vi "lab2_usrp_packet_transceiver.vi"() -> ()   [LabVIEW 2014]
uses:
  <vilib>/addons/Modulation/Analog/support/mod_Set Error Source.vi
  var_stop.vi
  <vilib>/addons/Modulation/Digital/Support/Common/Validators/mod_Generate Filter Coefficients Validate.vi
  <vilib>/addons/Modulation/Digital/General/subVIs/mod_Generate Filter Coefficients.vi
  <vilib>/measure/maspectr.llb/FFT Power Spectrum and PSD for 1 Chan (CDB).vi
  <vilib>/addons/Modulation/Digital/General/MT Apply Matched Filter (Generic).vi
  <vilib>/addons/Modulation/Digital/General/MT Align to Ideal Symbols (Generic).vi
  <instrlib>/niUSRP/niUSRP Fetch Rx Data (CDB Cluster).vi
  <instrlib>/niUSRP/niUSRP Write Tx Data (CDB Cluster).vi
  <vilib>/addons/Modulation/Digital/General/MT Apply Pulse Shaping Filter (Generic).vi
  <vilib>/addons/Modulation/niDMT.lvlib
  <vilib>/measure/NI_MAPro.lvlib
panel:
  out "ser/ber":dbl
  out "received symbols":u32
  out "error symbols":i16
  out "ser":dbl
  out "size2":i32
  out "size1":i32
  out "ber":dbl
  out "received bits":i32
  out "error bits":i16
  out "found?":bool
  out "# elements in queue":i32
  out "Spectrum monitor":cluster{"f0":dbl, "df":dbl, "magnitude":dbl[]}(graph)={"f0"=-0.49993781867926873, "df"=0.00012436264146250465, "magnitude"=[]}
  out "RX Constellation Map":cdb[](graph)
  out "valid?":bool
  in  "Gray code?":bool
  in  "Modulation":enum16{"PSK", "QAM"}(ring)=enum."QAM"
  out "Rx String":string
  in  "String":string
  out "packet len":u32
  in  "Send":bool
  in  "filter length (symbols)":i32=8
  in  "filter parameter":dbl=0.5 format="%.2f"
  in  "pulse shaping filter (none)":T1(ring)=enum."Raised Cosine"
  in  "M-PSK (4)":i32=16 caption="M-ARY"
  in  "samples per symbol (16)":i32=4
  out "packet bits length":i32
  in  "number of samples":i64=40000
  out "RX coerced gain":dbl format="%#_6f"
  out "RX coerced carrier frequency":dbl=915000000.0 format="%#_6p"
  out "RX coerced IQ rate":dbl=4000000.0 format="%#_6p"
  in  "RX active antenna":string="RX2"
  in  "RX gain":dbl format="%#_6f"
  in  "RX device names":refnum<k15>="192.168.10.2"
  out "TX coerced gain":dbl format="%#_6f"
  out "TX coerced carrier frequency":dbl=915000000.0 format="%#_6p"
  out "coerced IQ rate":dbl=4000000.0 format="%#_6p"
  in  "TX device names":refnum<k15>="192.168.10.2"
  in  "TX gain":dbl format="%#_6f"
  in  "carrier frequency":dbl=915000000.0 format="%#_6p"
  in  "IQ rate":dbl=800000.0 format="%#_6p"
  in  "stop":bool
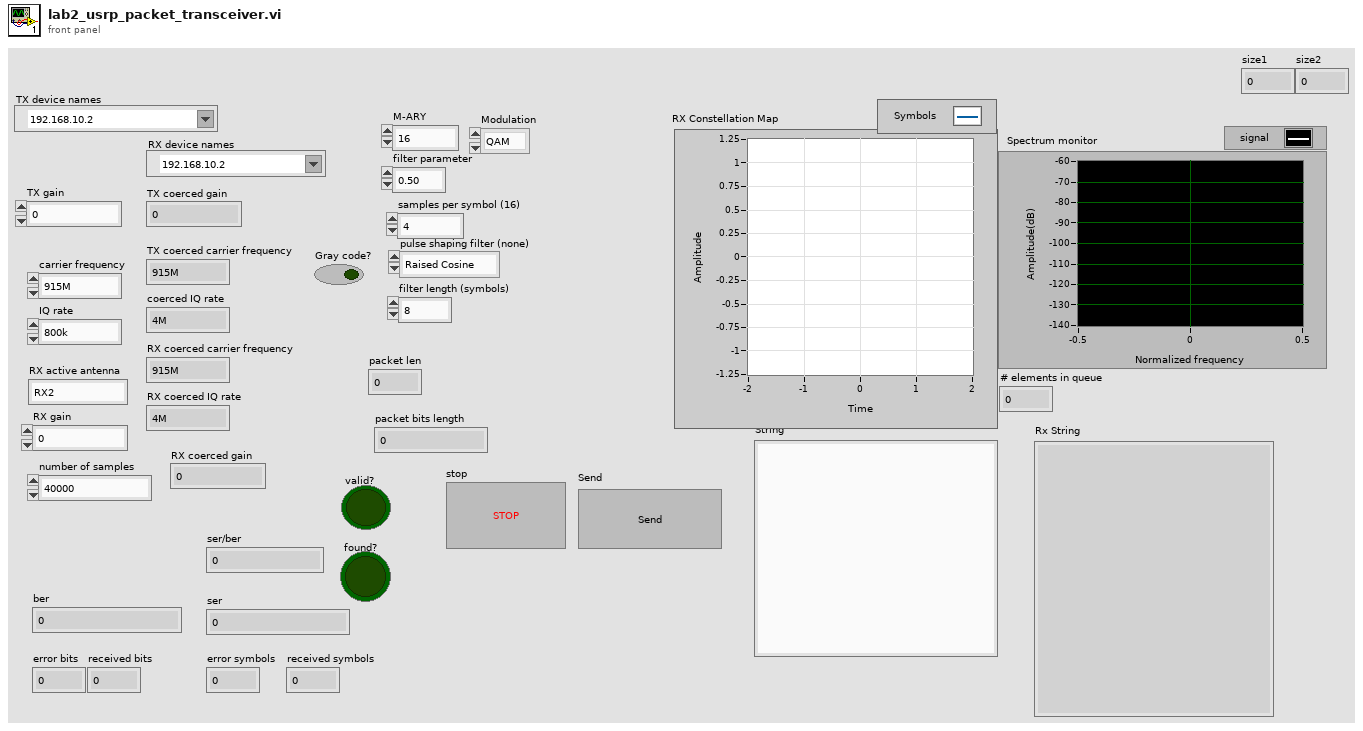
[diagram p1: front panel]
types:
  T1 = enum16{"none", "Raised Cosine", "Root Raised Cos", "Gaussian"}
  T2 = enum16{"FSK", "PSK", "QAM", "MSK", "PAM", "ASK", "CPM"}
  T3 = cluster{"samples per symbol (16)":i32, "symbol map":cdb[], "index map":u32[]}
  T4 = cluster{"samples per symbol (16)":i32, "symbol map":cdb[], i32[]}
  T5 = typedef "niAMT.lvlib/Complex Data Waveform.ctl" = cluster{"t0":dbl, "dt":dbl, "Y":cdb[]}
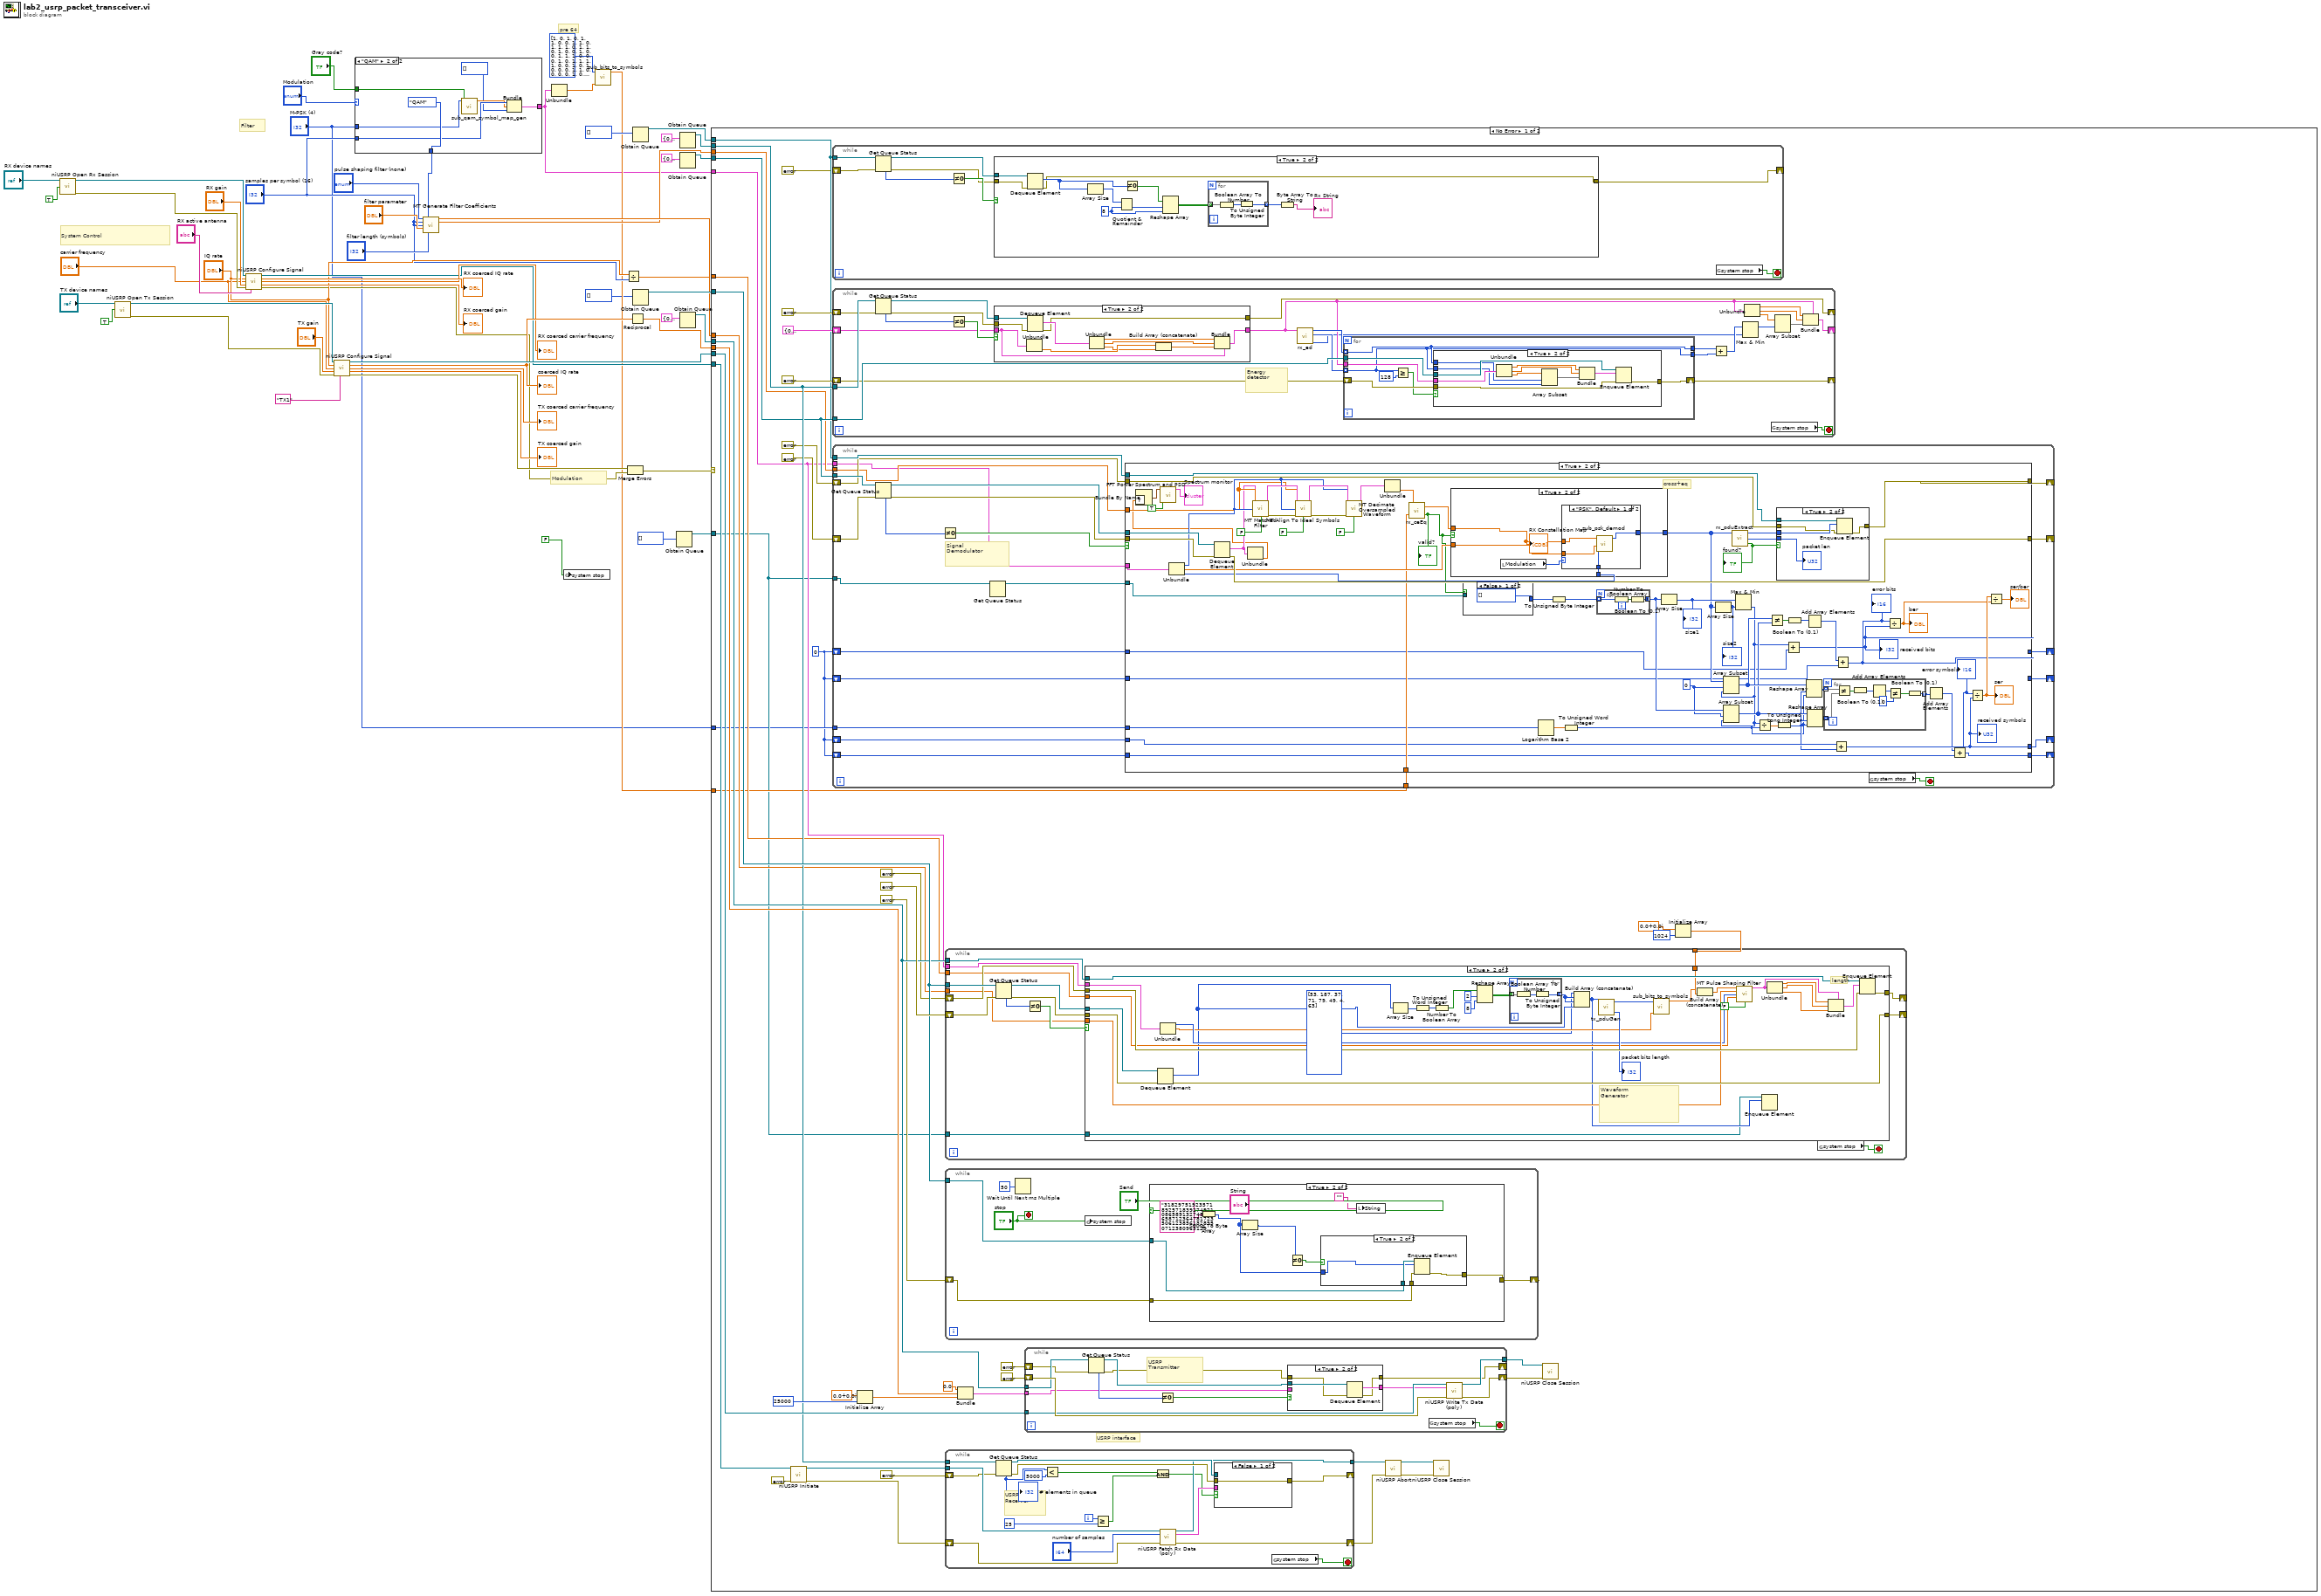
[diagram p0: block diagram]
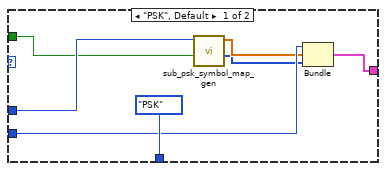
[diagram p2: hidden frame]
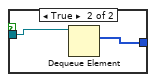
[diagram p5: hidden frame]
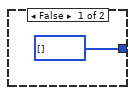
[diagram p6: hidden frame]
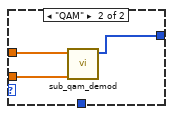
[diagram p7: hidden frame]
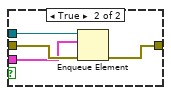
[diagram p11: hidden frame]
diagram:
  # "pre 64"
  # "Modulation"
  # "Filter"
  # "System Control"
  n1 = call <instrlib>:"niUSRP Open Rx Session.vi"("device names"="RX device names", "reset"=TRUE) -> ("session handle out"=w40:refnum<k15>, "error out"=w39:errorcluster)  [unwired: 12 in]
  n2 = call <instrlib>:"niUSRP Open Tx Session.vi"("device names"="TX device names", "reset"=TRUE) -> ("session handle out"=w53:refnum<k15>, "error out"=w52:errorcluster)  [unwired: 12 in]
  n3 = call <instrlib>:"niUSRP Configure Signal.vi"("session handle"=w40, "IQ rate"="IQ rate", "carrier frequency"="carrier frequency", "gain"="RX gain", "error in (no error)"=w39, "active antenna"="RX active antenna") -> ("session handle out"=w31:refnum<k15>, "coerced IQ rate"=→"RX coerced IQ rate":dbl, "coerced carrier frequency"=→"RX coerced carrier frequency":dbl, "coerced gain"=→"RX coerced gain":dbl, "error out"=w15:errorcluster)  [unwired: 5 in]
  n4 = call <instrlib>:"niUSRP Configure Signal.vi"("session handle"=w53, "IQ rate"="IQ rate", "carrier frequency"="carrier frequency", "gain"="TX gain", "error in (no error)"=w52, "active antenna"="TX1") -> ("session handle out"=w44:refnum<k15>, "coerced IQ rate"=w42:dbl, "coerced carrier frequency"=→"TX coerced carrier frequency":dbl, "coerced gain"=→"TX coerced gain":dbl, "error out"=w16:errorcluster)  [unwired: 5 in]
  "coerced IQ rate" <- w42
  n5 = case shown="\"QAM\"" "Modulation" {
    tunnel: [T2."PSK" ("modulation type") T2."QAM" ("modulation type")] -> w11
    tunnel: "M-PSK (4)" -> [w60 w66]
    tunnel: "Gray code?" -> [w59 w67]
    tunnel: "samples per symbol (16)" -> [w58 w65]
    tunnel: [w55 w62] -> w5
    frame "PSK", Default {
      n6 = call "sub_psk_symbol_map_gen.vi"("Gray code?"=w59, "M-PSK"=w60) -> ("index map"=w56:u32[], "symbol map"=w57:cdb[])  [unwired: 8 in]
      n7 = Bundle("samples per symbol (16)"=w58, "symbol map"=w57, "index map"=w56) -> (w55:T3)  [unwired: 1 in]
    }
    frame "QAM" {
      n8 = call "sub_qam_symbol_map_gen.vi"("Gray code?"=w67, "M-QAM"=w66) -> ("symbol map"=w64:cdb[])  [unwired: 9 in]
      n9 = Bundle("samples per symbol (16)"=w65, "symbol map"=w64, i32[] []) -> (w62:T4)  [unwired: 1 in]
    }
  }
  n10 = call <vilib>:"MT Generate Filter Coefficients.vi"("pulse shaping filter (none)"="pulse shaping filter (none)", "modulation type"=w11, "pulse shaping samples per symbol (16)"="samples per symbol (16)", "matched samples per symbol (16)"="samples per symbol (16)", "filter parameter"="filter parameter", "filter length (symbols)"="filter length (symbols)") -> ("pulse shaping filter coefficients"=w21:dbl[], "matched filter coefficients"=w19:dbl[])  [unwired: 7 in, 1 out]
  n11 = Unbundle(w5) -> ("symbol map"=w7:cdb[])  [unwired: 2 out]
  n12 = global write "var_stop.vi" "system stop"(FALSE) -> ()
  n13 = call "sub_bits_to_symbols.vi"("symbol map"=w7, "bits"=i16[] [1, 0, 1, 0, 1, 1, 0, 0, 1, 1, 0, 1, 1, 1, 0, 1, 1, 0, 1, 0, 0, 1, 0, 0, 1, 1, 1, 0, 0, 0, 1, 0, 1, 1, 1, 1, 0, 0, 1, 0, 1, 0, 0, 0, 1, 1, 0, 0, 0, 0, 1, 0, 0, 0, 0, 0, 1, 1, 1, 1, 1, 1, 0, 0] ("preamble(64) 2")) -> ("symbols"=w6:cdb[])  [unwired: 9 in]
  n14 = Divide(x="IQ rate", y="samples per symbol (16)") -> (x/y=w20:dbl)
  n15 = Merge Errors(w16, w15) -> (w14:errorcluster)
  n16 = Reciprocal(x=w42) -> (1/x=w41:dbl)
  n17 = Obtain Queue(element data type=i8[] [] ("output bit stream")) -> (queue out=w26:refnum<queue>)  [unwired: 4 in, 2 out]
  n18 = Obtain Queue(element data type=i16[] []) -> (queue out=w54:refnum<queue>)  [unwired: 4 in, 2 out]
  n19 = Obtain Queue(element data type=i16[] []) -> (queue out=w2:refnum<queue>)  [unwired: 4 in, 2 out]
  n20 = Obtain Queue(element data type=cluster{"t0":dbl, "dt":dbl, "Y":cdb[]} {"t0"=0.0, "dt"=0.0, "Y"=[]} ("data")) -> (queue out=w30:refnum<queue>)  [unwired: 4 in, 2 out]
  n21 = Obtain Queue(element data type=cluster{"t0":dbl, "dt":dbl, "Y":cdb[]} {"t0"=0.0, "dt"=0.0, "Y"=[]} ("data")) -> (queue out=w27:refnum<queue>)  [unwired: 4 in, 2 out]
  n22 = Obtain Queue(element data type=cluster{"t0":dbl, "dt":dbl, "Y":cdb[]} {"t0"=0.0, "dt"=1.0, "Y"=[]} ("data")) -> (queue out=w45:refnum<queue>)  [unwired: 4 in, 2 out]
  n23 = case shown="No Error" w14 {
    tunnel: w54 -> [w112 _]
    tunnel: w45 -> [w107 _]
    tunnel: w44 -> [w108 _]
    tunnel: w41 -> [w101 _]
    tunnel: w31 -> [w96 _]
    tunnel: w30 -> [w90 _]
    tunnel: w27 -> [w86 _]
    tunnel: w26 -> [w84 _]
    tunnel: w5 -> [w78 _]
    tunnel: w21 -> [w81 _]
    tunnel: w20 -> [w80 _]
    tunnel: w19 -> [w79 _]
    tunnel: w6 -> [w72 _]
    tunnel: w2 -> [w71 _]
    tunnel: "M-PSK (4)" -> [w70 _]
    frame No Error {
      w69 = 0
      # "USRP interface"
      n24 = call <instrlib>:"niUSRP Initiate.vi"("session handle"=w96, "error in (no error)"=errorcluster {"status"=FALSE, "code"=0, "source"=""}) -> ("session handle out"=w95:refnum<k15>, "error out"=w94:errorcluster)  [unwired: 12 in]
      n25 = while {
        tunnel: w84 -> [w121]
        shift-right: [w114] -> _
        shift-left: errorcluster {"status"=FALSE, "code"=0, "source"=""} ("error out") -> [w120]
        stop <- w119 stop-if-true
        n26 = Get Queue Status(queue=w121, error in (no error)=w120) -> (queue out=w116:refnum<queue>, error out=w115:errorcluster, # elements in queue=w118:i32)  [unwired: 1 in, 5 out]
        n27 = Not Equal To 0?(x=w118) -> (x != 0?=w117:bool)
        n28 = case shown="True" w117 {
          tunnel: w116 -> [_ w133]
          tunnel: w115 -> [w122 w132]
          tunnel: [w122 w125] -> w114
          frame False {
          }
          frame True {
            w128 = 8 ("y")
            n29 = Dequeue Element(queue=w133, error in (no error)=w132) -> (element=w131:i8[], error out=w125:errorcluster)  [unwired: 1 in, 2 out]
            n30 = Array Size(array=w131) -> (size(s)=w130:i32)
            n31 = Quotient & Remainder(x=w130, y=w128) -> (floor(x/y)=w127:i32)  [unwired: 1 out]
            n32 = Not Equal To 0?(x=w131) -> (x != 0?=w129:bool[])
            n33 = Reshape Array(w129, w127, w128) -> (w126:bool[][])
            n34 = for {
              tunnel: w126 -> [w136] mode=indexing
              tunnel: [w135] -> w124 mode=indexing
              n35 = Boolean Array To Number(Boolean array=w136) -> (number=w134:u32)
              n36 = To Unsigned Byte Integer(number=w134) -> (unsigned 8bit integer=w135:u8)
            }
            n37 = Byte Array To String(unsigned byte array=w124) -> (string=→"Rx String":string)
          }
        }
        n38 = global read "var_stop.vi" "system stop"() -> (w119:bool)
      }
      n39 = while {
        tunnel: w90 -> [w290]
        shift-right: [w283] -> _
        shift-left: errorcluster {"status"=FALSE, "code"=0, "source"=""} ("error out") -> [w289]
        shift-right: [w269] -> _
        shift-left: cluster{"t0":dbl, "dt":dbl, "Y":cdb[]} {"t0"=0.0, "dt"=0.0, "Y"=[]} ("data") -> [w284]
        tunnel: w86 -> [w282]
        shift-right: [w281] -> _
        shift-left: errorcluster {"status"=FALSE, "code"=0, "source"=""} ("error out") -> [w280]
        stop <- w279 stop-if-true
        # "Energy\ndetector"
        n40 = Get Queue Status(queue=w290, error in (no error)=w289) -> (queue out=w285:refnum<queue>, error out=w286:errorcluster, # elements in queue=w288:i32)  [unwired: 1 in, 5 out]
        n41 = Not Equal To 0?(x=w288) -> (x != 0?=w287:bool)
        n42 = case shown="True" w287 {
          tunnel: w286 -> [w312 w323]
          tunnel: w285 -> [_ w322]
          tunnel: w284 -> [w311 w317]
          tunnel: [w312 w314] -> w283
          tunnel: [w311 w313] -> w276
          frame False {
          }
          frame True {
            n43 = Unbundle(w317) -> ("Y"=w320:cdb[])  [unwired: 2 out]
            n44 = Dequeue Element(queue=w322, error in (no error)=w323) -> (element=w321:cluster{"t0":dbl, "dt":dbl, "Y":cdb[]}, error out=w314:errorcluster)  [unwired: 1 in, 2 out]
            n45 = Unbundle(w321) -> ("t0"=w316:dbl, "dt"=w315:dbl, "Y"=w319:cdb[])
            n46 = Build Array (concatenate)(w320, w319) -> (w318:cdb[])
            n47 = Bundle(cluster=w317, "t0"=w316, "dt"=w315, "Y"=w318) -> (w313:cluster{"t0":dbl, "dt":dbl, "Y":cdb[]})
          }
        }
        n48 = call "rx_ed.vi"("Wavefrom"=w276) -> ("first pulse"=w266:i32, "length"=w277:i32[], "start index"=w278:i32[])  [unwired: 8 in]
        n49 = for {
          tunnel: w282 -> [w298]
          tunnel: w276 -> [w295]
          shift-right: [w297] -> w281
          shift-left: w280 -> [w296]
          tunnel: w278 -> [w294] mode=indexing
          tunnel: w277 -> [w293] mode=indexing
          tunnel: [w294] -> w272
          tunnel: [w293] -> w271
          n50 = Greater Or Equal?(x=w293, y=128) -> (x >= y?=w291:bool)
          n51 = case shown="True" w291 {
            tunnel: w298 -> [_ w310]
            tunnel: [w299 w309] -> w297
            tunnel: w296 -> [w299 w308]
            tunnel: w295 -> [_ w307]
            tunnel: w294 -> [_ w301]
            tunnel: w293 -> [_ w300]
            frame False {
            }
            frame True {
              n52 = Unbundle(w307) -> ("t0"=w305:dbl, "dt"=w306:dbl, "Y"=w303:cdb[])
              n53 = Array Subset(array=w303, index=w301, length=w300) -> (w302:cdb[])
              n54 = Bundle("t0"=w305, "dt"=w306, w302) -> (w304:cluster{"t0":dbl, "dt":dbl, cdb[]})  [unwired: 1 in]
              n55 = Enqueue Element(queue=w310, element=w304, error in (no error)=w308) -> (error out=w309:errorcluster)  [unwired: 1 in, 2 out]
            }
          }
        }
        n56 = Add(x=w272, y=w271) -> (x+y=w268:i32)
        n57 = Max & Min(x=w268, y=w266) -> (max(x,y)=w267:i32)  [unwired: 1 out]
        n58 = Unbundle(w276) -> ("t0"=w275:dbl, "dt"=w274:dbl, "Y"=w273:cdb[])
        n59 = global read "var_stop.vi" "system stop"() -> (w279:bool)
        n60 = Array Subset(array=w273, index=w267) -> (w270:cdb[])  [unwired: 1 in]
        n61 = Bundle(cluster=w276, "t0"=w275, "dt"=w274, "Y"=w270) -> (w269:cluster{"t0":dbl, "dt":dbl, "Y":cdb[]})
      }
      n62 = while {
        tunnel: w86 -> [w161]
        shift-right: [w155] -> _
        shift-left: errorcluster {"status"=FALSE, "code"=0, "source"=""} ("error out") -> [w160]
        tunnel: w84 -> [w154]
        shift-right: [w153] -> _
        shift-left: errorcluster {"status"=FALSE, "code"=0, "source"=""} ("error out") -> [w152]
        tunnel: w79 -> [w150]
        tunnel: w78 -> [w149]
        tunnel: w72 -> [w148]
        tunnel: w71 -> [w147]
        tunnel: w70 -> [w145]
        shift-right: [w142] -> _
        shift-left: w69 -> [w144]
        shift-right: [w141] -> _
        shift-left: w69 -> [w143]
        shift-right: [w139] -> _
        shift-left: w69 -> [w140]
        shift-right: [w137] -> _
        shift-left: w69 -> [w138]
        stop <- w151 stop-if-true
        # "Signal \nDemodulator"
        n63 = Get Queue Status(queue=w161, error in (no error)=w160) -> (queue out=w157:refnum<queue>, error out=w156:errorcluster, # elements in queue=w159:i32)  [unwired: 1 in, 5 out]
        n64 = Not Equal To 0?(x=w159) -> (x != 0?=w158:bool)
        n65 = Get Queue Status(queue=w147) -> (queue out=w146:refnum<queue>)  [unwired: 2 in, 7 out]
        n66 = case shown="True" w158 {
          tunnel: w157 -> [_ w231]
          tunnel: w156 -> [w167 w232]
          tunnel: [w167 w230] -> w155
          tunnel: w154 -> [_ w221]
          tunnel: [w166 w220] -> w153
          tunnel: w152 -> [w166 w219]
          tunnel: w150 -> [_ w209]
          tunnel: w149 -> [_ w213]
          tunnel: w148 -> [_ w205]
          tunnel: w146 -> [_ w173]
          tunnel: w145 -> [_ w170]
          tunnel: w144 -> [w165 w184]
          tunnel: w143 -> [w164 w183]
          tunnel: [w165 w174] -> w142
          tunnel: [w164 w181] -> w141
          tunnel: w140 -> [w163 w180]
          tunnel: [w163 w178] -> w139
          tunnel: w138 -> [w162 w177]
          tunnel: [w162 w175] -> w137
          frame False {
          }
          frame True {
            w197 = 0
            # "cross+eq"
            n67 = Unbundle(w213) -> ("samples per symbol (16)"=w212:i32, "symbol map"=w211:cdb[], "index map"=w210:u32[])
            n68 = Dequeue Element(queue=w231, error in (no error)=w232) -> (element=w204:cluster{"t0":dbl, "dt":dbl, "Y":cdb[]}, error out=w230:errorcluster)  [unwired: 1 in, 2 out]
            n69 = Unbundle(w204) -> ("Y"=w203:cdb[])  [unwired: 2 out]
            n70 = Bundle By Name("Y"=w203) -> (w208:waveform(cdb))  [unwired: 1 in]
            n71 = call-poly <vilib>:"FFT Power Spectrum and PSD.vi"("dB On (F)"=TRUE, "time signal"=w208) -> ("Power Spectrum / PSD"=→"Spectrum monitor":cluster{"f0":dbl, "df":dbl, "magnitude":dbl[]})  [unwired: 6 in, 3 out]
            n72 = call-poly <vilib>:"MT Matched Filter.vi"("input complex waveform"=w204, "matched filter coefficients"=w209, "samples per symbol (16)"=w212, "reset? (T)"=FALSE) -> ("output complex waveform"=w229:T5, "error out"=w228:errorcluster)  [unwired: 10 in]
            n73 = call-poly <vilib>:"MT Align To Ideal Symbols.vi"("input complex waveform"=w229, "matched filter coefficients"=w209, "samples per symbol (16)"=w212, "error in (no error)"=w228, "reset? (T)"=FALSE) -> ("output complex waveform"=w226:T5, "error out"=w227:errorcluster)  [unwired: 8 in, 1 out]
            n74 = call <vilib>:"MT Decimate Oversampled Waveform.vi"("input complex waveform"=w226, "decimation factor"=w212, "error in (no error)"=w227, "reset? (T)"=FALSE) -> ("output complex waveform"=w225:T5)  [unwired: 10 in, 1 out]
            n75 = Unbundle(w225) -> ("Y"=w222:cdb[])  [unwired: 2 out]
            n76 = call "rx_ceEq.vi"("preamble"=w205, "symbols"=w222) -> ("valid?"=w171:bool, "eq symbols"=w218:cdb[])
            "valid?" <- w171
            n77 = case shown="True" w171 {
              tunnel: [i8[] [] ("output bit stream") w250] -> w199
              tunnel: w211 -> [_ w251]
              tunnel: w218 -> [_ w248]
              tunnel: w210 -> [_ w249]
              frame False {
              }
              frame True {
                n78 = local read "Modulation"() -> (w252:enum16{"PSK", "QAM"})
                n79 = case shown="\"PSK\", Default" w252 {
                  tunnel: w248 -> [w256 w259]
                  tunnel: w251 -> [w255 w258]
                  tunnel: [w253 w257] -> w250
                  tunnel: w249 -> [w254 _]
                  frame "PSK", Default {
                    n80 = call "sub_psk_demod.vi"("index map"=w254, "symbol map"=w255, "symbol"=w256) -> ("bitstream"=w253:i16[])  [unwired: 8 in]
                  }
                  frame "QAM" {
                    n81 = call "sub_qam_demod.vi"("symbol map"=w258, "symbol"=w259) -> ("bitstream"=w257:i16[])  [unwired: 9 in]
                  }
                }
                "RX Constellation Map" <- w248
              }
            }
            n82 = case shown="False" w171 {
              tunnel: w173 -> [_ w235]
              tunnel: [u16[] [] w234] -> w172
              frame False {
              }
              frame True {
                n83 = Dequeue Element(queue=w235) -> (element=w234:i16[])  [unwired: 2 in, 3 out]
              }
            }
            n84 = Logarithm Base 2(1:w170) -> (0:w169:dbl)
            n85 = To Unsigned Byte Integer(number=w172) -> (unsigned 8bit integer=w200:u8[])
            n86 = To Unsigned Word Integer(number=w169) -> (unsigned 16bit integer=w168:u16)
            n87 = for {
              tunnel: w200 -> [w246] mode=indexing
              tunnel: [w244] -> w198 mode=concatenating
              n88 = Number To Boolean Array(number=w246) -> (Boolean array=w245:bool[])
              n89 = Boolean To (0,1)(Boolean=w245) -> (0, 1=w244:i16[])
            }
            n90 = Array Size(array=w198) -> (size(s)=w201:i32)
            "size1" <- w201
            n91 = Array Size(array=w199) -> (size(s)=w202:i32)
            "size2" <- w202
            n92 = call "rx_pduExtract.vi"("output bit stream"=w199) -> ("found?"=w224:bool, "packet len"=w217:u32, "ppdu"=w223:i8[])  [unwired: 2 in]
            "found?" <- w224
            n93 = Max & Min(x=w201, y=w202) -> (min(x,y)=w185:i32)  [unwired: 1 out]
            n94 = Array Subset(array=w199, index=w197, length=w185) -> (w194:i16[])
            n95 = Array Subset(array=w198, index=w197, length=w185) -> (w193:i16[])
            n96 = Divide(x=w185, y=w168) -> (x/y=w189:dbl)
            n97 = Not Equal?(x=w194, y=w193) -> (x != y?=w196:bool[])
            n98 = case shown="True" w224 {
              tunnel: w223 -> [_ w263]
              tunnel: w221 -> [_ w265]
              tunnel: [w260 w264] -> w220
              tunnel: w219 -> [w260 w261]
              tunnel: w217 -> [_ w262]
              frame False {
              }
              frame True {
                n99 = Enqueue Element(queue=w265, element=w263, error in (no error)=w261) -> (error out=w264:errorcluster)  [unwired: 1 in, 2 out]
                "packet len" <- w262
              }
            }
            n100 = To Unsigned Long Integer(number=w189) -> (unsigned 32bit integer=w179:u32)
            n101 = Add(x=w185, y=w184) -> (x+y=w174:i32)
            "received bits" <- w174
            n102 = Boolean To (0,1)(Boolean=w196) -> (0, 1=w195:i16[])
            n103 = Reshape Array(w194, w179, w168) -> (w192:i16[][])
            n104 = Add Array Elements(numeric array=w195) -> (sum=w182:i16)
            n105 = Reshape Array(w193, w179, w168) -> (w191:i16[][])
            n106 = for {
              tunnel: w192 -> [w238] mode=indexing
              tunnel: w191 -> [w237] mode=indexing
              tunnel: [w236] -> w190 mode=indexing
              n107 = Not Equal?(x=w238, y=w237) -> (x != y?=w243:bool[])
              n108 = Boolean To (0,1)(Boolean=w243) -> (0, 1=w242:i16[])
              n109 = Add Array Elements(numeric array=w242) -> (sum=w241:i16)
              n110 = Not Equal?(x=w241, y=0) -> (x != y?=w239:bool)
              n111 = Boolean To (0,1)(Boolean=w239) -> (0, 1=w236:i16)
            }
            n112 = Add(x=w180, y=w179) -> (x+y=w178:u32)
            "received symbols" <- w178
            n113 = Add(x=w182, y=w183) -> (x+y=w181:i32)
            "error bits" <- w181
            n114 = Divide(x=w181, y=w174) -> (x/y=w187:dbl)
            "ber" <- w187
            n115 = Add Array Elements(numeric array=w190) -> (sum=w176:i16)
            n116 = Add(x=w176, y=w177) -> (x+y=w175:i32)
            "error symbols" <- w175
            n117 = Divide(x=w175, y=w178) -> (x/y=w188:dbl)
            "ser" <- w188
            n118 = Divide(x=w188, y=w187) -> (x/y=→"ser/ber":dbl)
          }
        }
        n119 = global read "var_stop.vi" "system stop"() -> (w151:bool)
      }
      n120 = Initialize Array(cdb 0.0+0.0i, 25000 ("dimension size")) -> (w102:cdb[])
      n121 = while {
        tunnel: w112 -> [w425]
        shift-right: [w423] -> _
        shift-left: errorcluster {"status"=FALSE, "code"=0, "source"=""} ("error out") -> [w424]
        stop <- "stop" stop-if-true
        n122 = Wait Until Next ms Multiple(millisecond multiple=u32 50) -> ()  [unwired: 1 out]
        n123 = global write "var_stop.vi" "system stop"("stop") -> ()
        n124 = case shown="True" "Send" {
          tunnel: w425 -> [_ w433]
          tunnel: w424 -> [w428 w432]
          tunnel: [w428 w431] -> w423
          frame False {
          }
          frame True {
            n125 = String To Byte Array(string="318297519235718925718392749210865891327481326587123647817235061238561328950712380965129083740123658129379123658291374931829751923571892571839274921086589132748132658712364781723506123856132895071238096512908374012365812937912365829137493182975192357189257183927492108658913274813265871236478172350612385613289507123809651290837401236581293791236582913749") -> (unsigned byte array=w434:u8[])
            n126 = Array Size(array=w434) -> (size(s)=w430:i32)
            n127 = Not Equal To 0?(x=w430) -> (x != 0?=w435:bool)
            n128 = case shown="True" w435 {
              tunnel: w434 -> [_ w438]
              tunnel: w433 -> [_ w441]
              tunnel: w432 -> [w437 w440]
              tunnel: [w437 w439] -> w431
              frame False {
              }
              frame True {
                n129 = Enqueue Element(queue=w441, element=w438, error in (no error)=w440) -> (error out=w439:errorcluster)  [unwired: 1 in, 2 out]
              }
            }
            n130 = local write "String"("") -> ()
          }
        }
      }
      n131 = while {
        tunnel: w95 -> [w342]
        shift-right: [w330] -> w91
        shift-left: w94 -> [w341]
        tunnel: w90 -> [w339]
        shift-right: [w333] -> _
        shift-left: errorcluster {"status"=FALSE, "code"=0, "source"=""} ("error out") -> [w338]
        tunnel: [w331] -> w92
        i -> [w328]
        stop <- w329 stop-if-true
        # "USRP\nReceiver"
        n132 = Get Queue Status(queue=w339, error in (no error)=w338) -> (queue out=w335:refnum<queue>, error out=w334:errorcluster, # elements in queue=w337:i32)  [unwired: 1 in, 5 out]
        "# elements in queue" <- w337
        n133 = Less?(x=w337, y=5000) -> (x < y?=w326:bool)
        n134 = Greater Or Equal?(x=w328, y=25) -> (x >= y?=w325:bool)
        n135 = And(x=w326, y=w325) -> (x .and. y?=w324:bool)
        n136 = call-poly <instrlib>:"niUSRP Fetch Rx Data (poly).vi"("session handle"=w342, "number of samples"="number of samples", "error in (no error)"=w341) -> ("session handle out"=w331:refnum<k15>, "data"=w332:cluster{"t0":dbl, "dt":dbl, "Y":cdb[]}, "error out"=w330:errorcluster)  [unwired: 9 in, 1 out]
        n137 = case shown="False" w324 {
          tunnel: w335 -> [_ w347]
          tunnel: w334 -> [w343 w346]
          tunnel: [w343 w345] -> w333
          tunnel: w332 -> [_ w344]
          frame False {
          }
          frame True {
            n138 = Enqueue Element(queue=w347, element=w344, error in (no error)=w346) -> (error out=w345:errorcluster)  [unwired: 1 in, 2 out]
          }
        }
        n139 = global read "var_stop.vi" "system stop"() -> (w329:bool)
      }
      n140 = Bundle(0.0, w101, w102) -> (w99:cluster{dbl, dbl, cdb[]})  [unwired: 1 in]
      n141 = while {
        shift-right: [w357] -> w111
        shift-left: errorcluster {"status"=FALSE, "code"=0, "source"=""} ("error out") -> [w355]
        tunnel: [w356] -> w110
        tunnel: w108 -> [w354]
        tunnel: w107 -> [w352]
        shift-right: [w350] -> _
        shift-left: errorcluster {"status"=FALSE, "code"=0, "source"=""} ("error out") -> [w351]
        tunnel: w99 -> [w349]
        stop <- w348 stop-if-true
        # "USRP\nTransmitter"
        n142 = Get Queue Status(queue=w352, error in (no error)=w351) -> (queue out=w359:refnum<queue>, error out=w358:errorcluster, # elements in queue=w361:i32)  [unwired: 1 in, 5 out]
        n143 = Not Equal To 0?(x=w361) -> (x != 0?=w360:bool)
        n144 = case shown="True" w360 {
          tunnel: w359 -> [_ w367]
          tunnel: w358 -> [w362 w366]
          tunnel: [w363 w365] -> w353
          tunnel: [w362 w364] -> w350
          tunnel: w349 -> [w363 _]
          frame False {
          }
          frame True {
            n145 = Dequeue Element(queue=w367, error in (no error)=w366) -> (element=w365:cluster{"t0":dbl, "dt":dbl, "Y":cdb[]}, error out=w364:errorcluster)  [unwired: 1 in, 2 out]
          }
        }
        n146 = global read "var_stop.vi" "system stop"() -> (w348:bool)
        n147 = call-poly <instrlib>:"niUSRP Write Tx Data (poly).vi"("session handle"=w354, "data"=w353, "error in (no error)"=w355) -> ("session handle out"=w356:refnum<k15>, "error out"=w357:errorcluster)  [unwired: 11 in]
      }
      n148 = call <instrlib>:"niUSRP Abort.vi"("session handle"=w92, "error in (no error)"=w91) -> ("session handle out"=w98:refnum<k15>, "error out"=w97:errorcluster)  [unwired: 12 in]
      n149 = call <instrlib>:"niUSRP Close Session.vi"("session handle"=w98, "error in (no error)"=w97) -> ()  [unwired: 13 in, 1 out]
      n150 = call <instrlib>:"niUSRP Close Session.vi"("session handle"=w110, "error in (no error)"=w111) -> ()  [unwired: 13 in, 1 out]
      n151 = Initialize Array(cdb 0.0+0.0i, 1024 ("dimension size")) -> (w73:cdb[])
      n152 = while {
        tunnel: w112 -> [w380]
        shift-right: [w377] -> _
        shift-left: errorcluster {"status"=FALSE, "code"=0, "source"=""} ("error out") -> [w383]
        tunnel: w107 -> [w376]
        shift-right: [w375] -> _
        shift-left: errorcluster {"status"=FALSE, "code"=0, "source"=""} ("error out") -> [w374]
        tunnel: w78 -> [w372]
        tunnel: w81 -> [w371]
        tunnel: w80 -> [w370]
        tunnel: w73 -> [w369]
        tunnel: w71 -> [w368]
        stop <- w373 stop-if-true
        n153 = Get Queue Status(queue=w380, error in (no error)=w383) -> (queue out=w378:refnum<queue>, error out=w379:errorcluster, # elements in queue=w382:i32)  [unwired: 1 in, 5 out]
        n154 = Not Equal To 0?(x=w382) -> (x != 0?=w381:bool)
        n155 = case shown="True" w381 {
          tunnel: w379 -> [w385 w418]
          tunnel: w378 -> [_ w417]
          tunnel: [w385 w416] -> w377
          tunnel: w376 -> [_ w411]
          tunnel: [w384 w410] -> w375
          tunnel: w374 -> [w384 w409]
          tunnel: w372 -> [_ w407]
          tunnel: w371 -> [_ w406]
          tunnel: w370 -> [_ w405]
          tunnel: w369 -> [_ w395]
          tunnel: w368 -> [_ w386]
          frame False {
          }
          frame True {
            # "length"
            # "Waveform \nGenerator"
            n156 = Dequeue Element(queue=w417, error in (no error)=w418) -> (element=w391:i16[], error out=w416:errorcluster)  [unwired: 1 in, 2 out]
            n157 = Unbundle(w407) -> ("samples per symbol (16)"=w401:i32, "symbol map"=w393:cdb[])  [unwired: 1 out]
            n158 = Array Size(array=w391) -> (size(s)=w403:i32)
            n159 = To Unsigned Word Integer(number=w403) -> (unsigned 16bit integer=w402:u16)
            n160 = Number To Boolean Array(number=w402) -> (Boolean array=w415:bool[])
            n161 = Reshape Array(w415, 2 ("dimension size"), 8 ("dimension size")) -> (w412:bool[][])
            n162 = for {
              tunnel: w412 -> [w421] mode=indexing
              tunnel: [w419] -> w404 mode=indexing
              n163 = Boolean Array To Number(Boolean array=w421) -> (number=w420:u32)
              n164 = To Unsigned Byte Integer(number=w420) -> (unsigned 8bit integer=w419:u8)
            }
            n165 = Build Array (concatenate)(u8[] [53, 187, 37, 71, 79, 49, 4, 63] ("Array 2"), w404, w404, w391) -> (w387:i16[])
            n166 = call "tx_pduGen.vi"("byte array"=w387) -> ("packet bits length"=→"packet bits length":i32, "pdu"=w394:i32[])  [unwired: 3 in]
            n167 = call "sub_bits_to_symbols.vi"("symbol map"=w393, "bits"=w394) -> ("symbols"=w392:cdb[])  [unwired: 9 in]
            n168 = Build Array (concatenate)(w392, w395) -> (w388:cdb[])
            n169 = call-poly <vilib>:"MT Pulse Shaping Filter.vi"("symbols"=w388, "pulse shaping filter coefficients"=w406, "samples per symbol (16)"=w401, "symbol rate (Hz)"=w405, "reset? (T)"=FALSE) -> ("output complex waveform"=w400:T5)  [unwired: 9 in, 1 out]
            n170 = Enqueue Element(queue=w386, element=w387) -> ()  [unwired: 2 in, 3 out]
            n171 = Unbundle(w400) -> ("t0"=w399:dbl, "dt"=w398:dbl, "Y"=w390:cdb[])
            n172 = Bundle(cluster=w400, "t0"=w399, "dt"=w398, "Y"=w390) -> (w397:T5)
            n173 = Enqueue Element(queue=w411, element=w397, error in (no error)=w409) -> (error out=w410:errorcluster)  [unwired: 1 in, 2 out]
          }
        }
        n174 = global read "var_stop.vi" "system stop"() -> (w373:bool)
      }
    }
    frame Error {
    }
  }
